vi "Set Delimit.vi"(8 "error in (no error)":errorcluster caption="entrée d'erreur (pas d'erreur)", 10 "Delimit":string, 11 "Class Instrument Log_File en entrée":refnum<class "Class Instrument Log_File.lvclass">) -> (0 "error out":errorcluster caption="sortie d'erreur", 3 "Class Instrument Log_File en sortie":refnum<class "Class Instrument Log_File.lvclass">)   [LabVIEW 2020, in "Library Instrument & Equipement.lvlib" / "Library Instruments.lvlib" / "Class Instrument Log_File.lvclass"]
uses:
  Class Instrument Log_File.lvclass
  Class Instrument Log_File.lvclass/Class Instrument Log_File.ctl
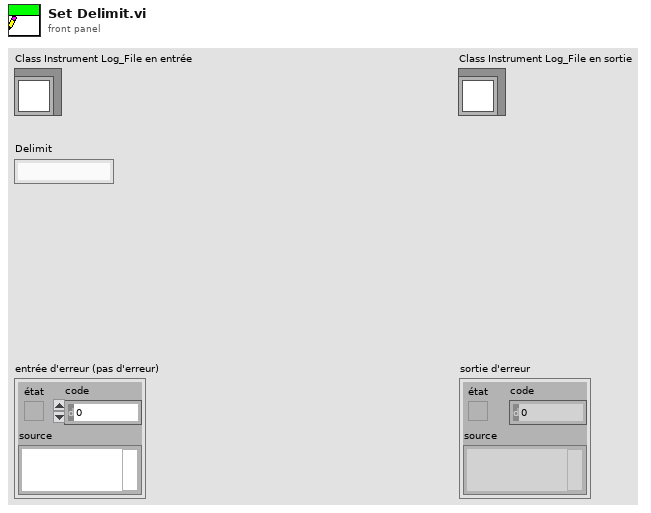
[diagram p1: front panel]
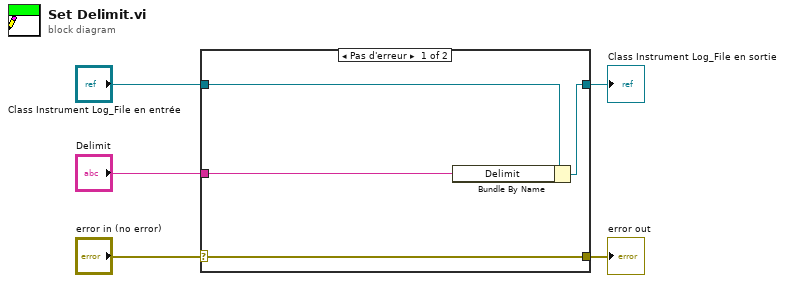
[diagram p0: block diagram]
diagram:
  n1 = case shown="Pas d'erreur" "error in (no error)" {
    selector: "error in (no error)" -> [w9 w10]
    tunnel: [w9 w10] -> w4
    tunnel: [w7 w11] -> w2
    tunnel: "Class Instrument Log_File en entrée" -> [w8 w11]
    tunnel: "Delimit" -> [w6 _]
    frame No Error {
      n2 = Bundle By Name(cluster=w8, "Delimit"=w6) -> (w7:refnum<class "Class Instrument Log_File.lvclass">)
    }
    frame Error {
    }
  }
  "error out" <- w4
  "Class Instrument Log_File en sortie" <- w2
